vi "P6.vi"() -> ()   [LabVIEW 2024]
panel:
  out "RTD, ohms":dbl format="%0#1.2f"
  out "Hot":bool
  out "Cold":bool
  in  "stop":bool
  out "Vp, mv":dbl format="%0#1.2g"
  out "Vdiff, mv":dbl format="%0#1.2f"
  out "Temp, C":dbl format="%0#1.1f"
  out "Waveform Chart":dbl(graph)
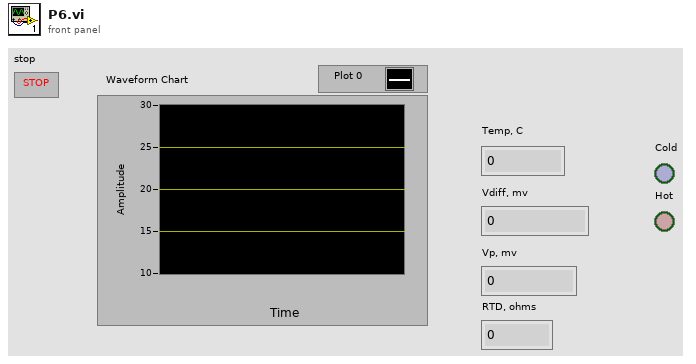
[diagram p1: front panel]
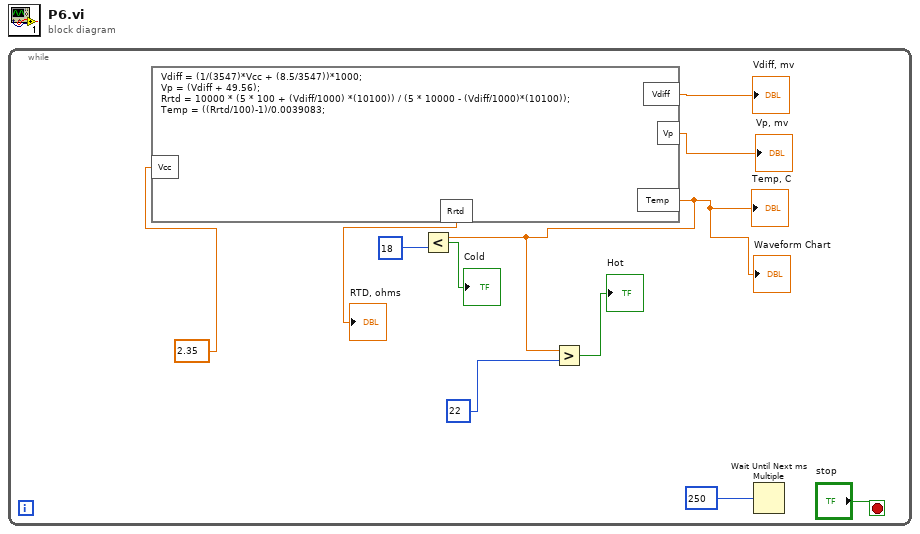
[diagram p0: block diagram]
diagram:
  n1 = while {
    stop <- "stop" stop-if-true
    n2 = formula code="Vdiff = (1/(3547)*Vcc + (8.5/3547))*1000;\nVp = (Vdiff + 49.56);\nRrtd = 10000 * (5 * 100 + (Vdiff/1000) *(10100)) / (5 * 10000 - (Vdiff/1000)*(10100));\nTemp = ((Rrtd/100)-1)/0.0039083;"("Vcc"=2.35) -> ("Vdiff"=→"Vdiff, mv":dbl, "Vp"=→"Vp, mv":dbl, "Temp"=w4:dbl, "Rrtd"=→"RTD, ohms":dbl)
    "Waveform Chart" <- w4
    "Temp, C" <- w4
    n3 = Less?(x=w4, y=18) -> (x < y?=→"Cold":bool)
    n4 = Greater?(x=w4, y=22) -> (0:→"Hot":bool)
    n5 = Wait Until Next ms Multiple(millisecond multiple=250) -> ()  [unwired: 1 out]
  }
